vi "ProvisioningSetEndpointAuthsRoutedMessage_Parse.vi"(8 "error in (no error)":errorcluster, 11 "Message":T5) -> (0 "error out":errorcluster, 1 "Body":T1, 2 "Header":T3, 3 "ProvisioningSetEndpointAuthsRoutedMessage":T2)   [LabVIEW 2017]
uses:
  <vilib>/addons/InsightCM/MessageBus/Base/controls/Message.ctl
  <vilib>/addons/InsightCM/MessageBus/Base/controls/MessageHeader.ctl
  <vilib>/addons/InsightCM/MessageBus/Base/controls/KeyValuePair.ctl
  <vilib>/addons/InsightCM/MessageBus/MessageLibrary/Provisioning/controls/ProvisioningSetEndpointAuthsRoutedMessage.ctl
  <vilib>/addons/InsightCM/MessageBus/MessageLibrary/Provisioning/controls/ProvisioningSetEndpointAuthsRoutedMessageBody.ctl
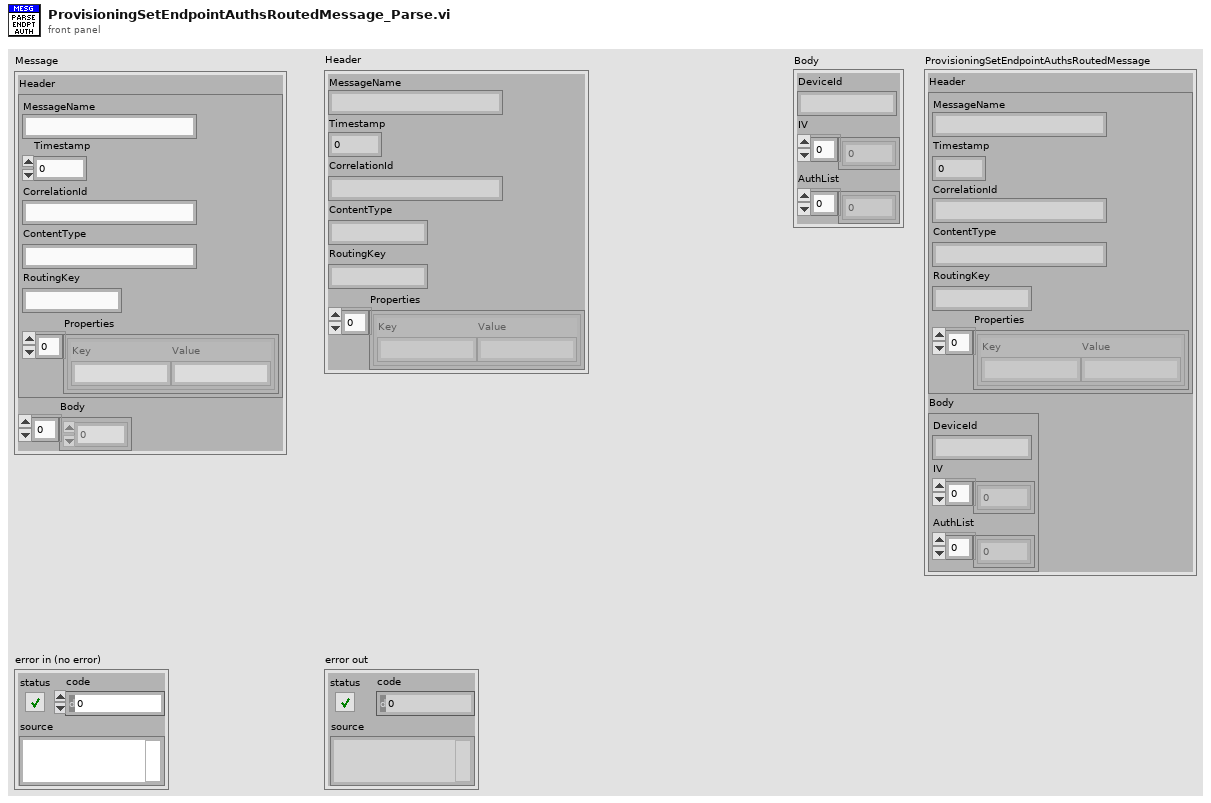
[diagram p1: front panel]
types:
  T1 = typedef "ProvisioningSetEndpointAuthsRoutedMessageBody.ctl" = cluster{"DeviceId":string, "IV":u8[], "AuthList":u8[]}
  T2 = typedef "ProvisioningSetEndpointAuthsRoutedMessage.ctl" = cluster{"Header":T3, "Body":T1}
  T3 = typedef "MessageHeader.ctl" = cluster{"MessageName":string, "Timestamp":i64, "CorrelationId":string, "ContentType":string, "RoutingKey":string, "Properties":T4[]}
  T4 = typedef "KeyValuePair.ctl" = cluster{"Key":string, "Value":string}
  T5 = typedef "Message.ctl" = cluster{"Header":T3, "Body":u8[]}
  T6 = cluster{"DeviceId":string, "IV":string, "AuthList":string}
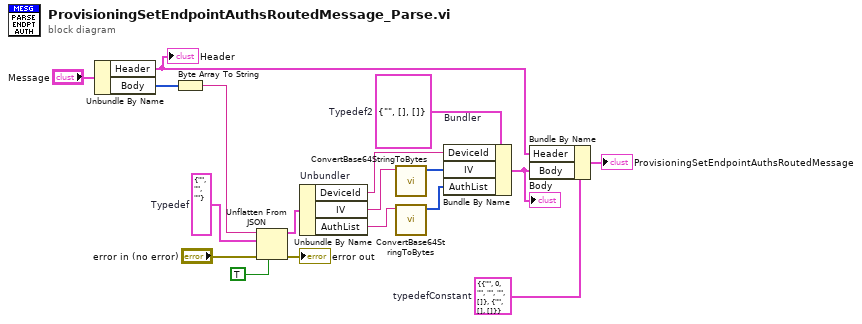
[diagram p0: block diagram]
diagram:
  w6 = T1 {"DeviceId"="", "IV"=[], "AuthList"=[]}  # Typedef2
  w10 = T2 {"Header"={"MessageName"="", "Timestamp"=0, "CorrelationId"="", "ContentType"="", "RoutingKey"="", "Properties"=[]}, "Body"={"DeviceId"="", "IV"=[], "AuthList"=[]}}  # typedefConstant
  w14 = T6 {"DeviceId"="", "IV"="", "AuthList"=""}  # Typedef
  n1 = Unbundle By Name("Message") -> ("Header"=w16:T3, "Body"=w8:u8[])
  "Header" <- w16
  n2 = Byte Array To String(unsigned byte array=w8) -> (string=w13:string)
  n3 = Unflatten From JSON(JSON string=w13, type and defaults=w14, default null elements? (F)=TRUE, error in (no error)="error in (no error)") -> (value=w12:T6, error out=→"error out":errorcluster)  [unwired: 3 in]
  n4 = Unbundle By Name "Unbundler"(w12) -> ("DeviceId"=w5:string, "IV"=w4:string, "AuthList"=w2:string)
  n5 = call <vilib>:"ConvertBase64StringToBytes.vi"("Base64 string"=w4) -> ("U8 array"=w3:u8[])  [unwired: 9 in, 1 out]
  n6 = call <vilib>:"ConvertBase64StringToBytes.vi"("Base64 string"=w2) -> ("U8 array"=w1:u8[])  [unwired: 9 in, 1 out]
  n7 = Bundle By Name "Bundler"(cluster=w6, "DeviceId"=w5, "IV"=w3, "AuthList"=w1) -> (w7:T1)
  "Body" <- w7
  n8 = Bundle By Name(cluster=w10, "Header"=w16, "Body"=w7) -> (→"ProvisioningSetEndpointAuthsRoutedMessage":T2)
